vi "StartCapture.vi"(8 "error in (no error)":errorcluster, 10 "Continuous":bool, 11 "ZWO_ASI in":refnum<class "ZWO_ASI.lvclass">) -> (0 "error out":errorcluster, 3 "ZWO_ASI out":refnum<class "ZWO_ASI.lvclass">)   [LabVIEW 2023, in "ZWO_ASI.lvlib" / "ZWO_ASI.lvclass"]
uses:
  ZWO_ASI.lvclass
  Labview_ASI_demo_64bit_221128/user.lib/ASICamera2_no_err/ASICamera2_no_err.lvlib
  ZWO_ASI Messages/GetFrame Msg/GetFrame Msg.lvclass
  <vilib>/ActorFramework/Actor/Actor.lvclass
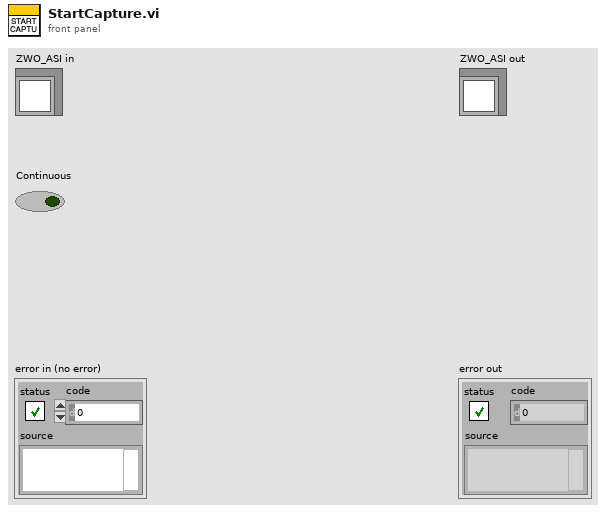
[diagram p1: front panel]
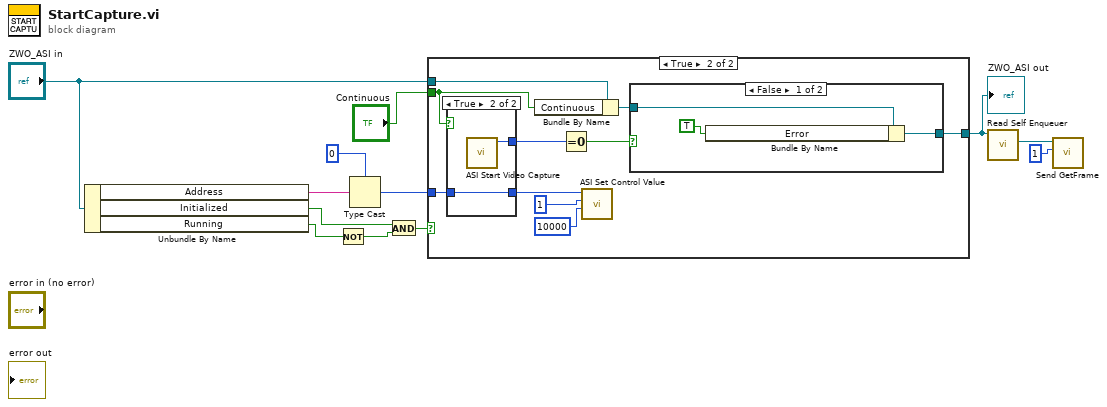
[diagram p0: block diagram]
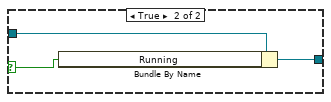
[diagram p3: hidden frame]
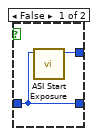
[diagram p4: hidden frame]
diagram:
  n1 = Unbundle By Name("ZWO_ASI in") -> ("Address"=w3:string, "Initialized"=w9:bool, "Running"=w11:bool)
  n2 = Not(x=w11) -> (.not. x?=w10:bool)
  n3 = Type Cast(type=0 ("iCameraID"), x=w3) -> (*(type *) &x=w2:i32)
  n4 = And(x=w9, y=w10) -> (x .and. y?=w8:bool)
  n5 = case shown="True" w8 {
    tunnel: "ZWO_ASI in" -> [w13 w15]
    tunnel: [w13 w21] -> w6
    tunnel: w2 -> [_ w20]
    tunnel: "Continuous" -> [_ w14]
    frame False {
    }
    frame True {
      n6 = case shown="True" w14 {
        tunnel: [w31 w33] -> w23
        tunnel: w20 -> [w30 w32]
        tunnel: [w30 w32] -> w19
        frame False {
          n7 = call "ASI Start Exposure.vi"("iCameraID"=w30) -> ("function return"=w31:i32)  [unwired: 10 in]
        }
        frame True {
          n8 = call "ASI Start Video Capture.vi"() -> ("function return"=w33:i32)  [unwired: 11 in]
        }
      }
      n9 = Bundle By Name(cluster=w15, "Continuous"=w14) -> (w16:refnum<class "ZWO_ASI.lvclass">)
      n10 = Equal To 0?(x=w23) -> (x = 0?=w22:bool)
      n11 = call "ASI Set Control Value.vi"("lValue"=10000, "ControlType"=1, "iCameraID"=w19) -> ()  [unwired: 8 in, 1 out]
      n12 = case shown="False" w22 {
        selector: w22 -> [_ w28]
        tunnel: w16 -> [w26 w29]
        tunnel: [w25 w27] -> w21
        frame False {
          n13 = Bundle By Name(cluster=w26, "Error"=TRUE) -> (w25:refnum<class "ZWO_ASI.lvclass">)
        }
        frame True {
          n14 = Bundle By Name(cluster=w29, "Running"=w28) -> (w27:refnum<class "ZWO_ASI.lvclass">)
        }
      }
    }
  }
  "ZWO_ASI out" <- w6
  n15 = call <vilib>:"Read Self Enqueuer.vi"("Actor"=w6) -> ("Self Enqueuer"=w7:refnum<class "Message Enqueuer.lvclass">)  [unwired: 10 in]
  n16 = call "Send GetFrame.vi"("num of frames"=1, "Message Enqueuer"=w7) -> ()  [unwired: 8 in, 2 out]
